vi "Write Config.vi"(8 "error in (no error)":errorcluster, 9 "Re-Init?":bool, 10 "ICM File In":path, 11 "Multi Parser in":refnum<class "Mulit Sentence Parser.lvclass">) -> (0 "error out":errorcluster, 3 "Multi Parser out":refnum<class "Mulit Sentence Parser.lvclass">)   [LabVIEW 2015, in "Mulit Sentence Parser.lvclass"]
doc: "Multi Sentence Parser.lvclass:Write Config.vi\n\nThis VI writes the Multi Sentence Parser Class parameters to the ICM configuration file.\n\nInstrument Communication Module Version 1.0\nOctober, 2018 Original Code Consulting David Thomson\n www.originalcode.com"
uses:
  Mulit Sentence Parser.lvclass
  Mulit Sentence Parser.lvclass/Mulit Sentence Parser.ctl
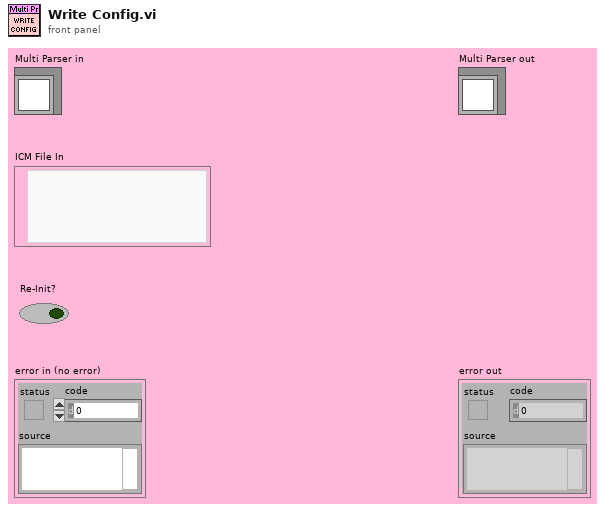
[diagram p1: front panel]
types:
  T1 = typedef "Mulit Sentence Parser.lvclass/Multi Sentence Parser Config.ctl" = cluster{"Sentences":cluster{"Sentence ID":string, "Format String":string, "Channels":string[], "Enabled":bool[]}[]}
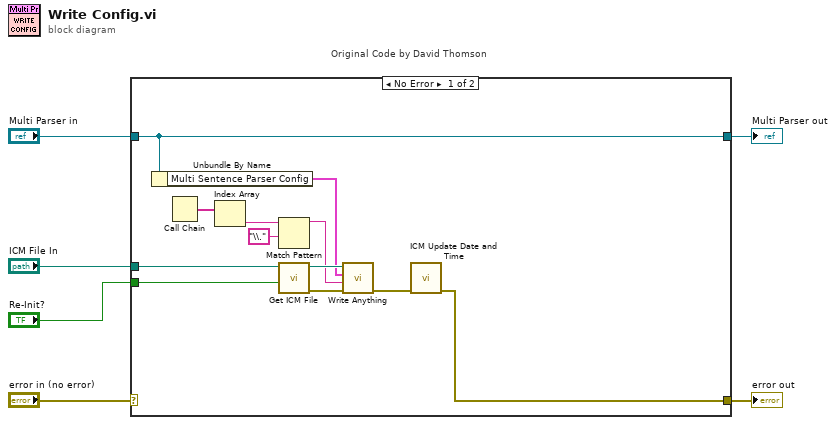
[diagram p0: block diagram]
diagram:
  n1 = case "Original Code by David Thomson" shown="No Error" "error in (no error)" {
    selector: "error in (no error)" -> [_ w20]
    tunnel: [w9 w20] -> w5
    tunnel: [w8 w19] -> w3
    tunnel: "Multi Parser in" -> [w8 w19]
    tunnel: "ICM File In" -> [w12 _]
    tunnel: "Re-Init?" -> [w11 _]
    frame No Error {
      n2 = Unbundle By Name(w8) -> ("Multi Sentence Parser Config"=w7:T1)
      n3 = Call Chain() -> (call chain=w17:string[])
      n4 = Index Array(array=w17) -> (element=w16:string)  [unwired: 1 in]
      n5 = Match Pattern(string=w16, regular expression="\\.") -> (before substring=w13:string)  [unwired: 1 in, 3 out]
      n6 = call "Get ICM File.vi"("Re-Init?"=w11, "ICM File In"=w12) -> ("error out"=w15:errorcluster, "ICM File"=w14:path)  [unwired: 8 in]
      n7 = call "Write Anything.vi"("Error In"=w15, "Section Name (Name of \"Anything\")"=w13, "Anything"=w7, "Path (dialog)"=w14) -> ("Error Out"=w10:errorcluster)  [unwired: 7 in]
      n8 = call "ICM Update Date and Time.vi"("error in (no error)"=w10) -> ("error out"=w9:errorcluster)  [unwired: 9 in, 1 out]
    }
    frame Error {
    }
  }
  "error out" <- w5
  "Multi Parser out" <- w3
